vi "Duplicate.vi"(8 "error in":errorcluster, 10 "parameters":variant, 11 "DMM Instrument in":refnum<class "DMM Instrument.lvclass">) -> (0 "error out":errorcluster, 3 "DMM Instrument out":refnum<class "DMM Instrument.lvclass">)   [LabVIEW 2025, in "DMM.lvlib" / "DMM Instrument.lvclass"]
doc: "Implements the specific behavior of a node when it is being duplicated\nCan be used to change the name of the new node for example adding Copy to it. \nCopyright 2017 National Instruments Corporation\n\nLicensed under the Apache License, Version 2.0 (the \"License\"); you may not use this file except in compliance with the License. You may obtain a copy of the License at http://www.apache.org/licenses/LICENSE-2.0\nUnless required by applicable law or agreed to in writing, software distributed under the License is distributed on an \"AS IS\" BASIS, WITHOUT WARRANTIES OR CONDITIONS OF ANY KIND, either express or implied. See the License for the specific language governing permissions and limitations under the License."
uses:
  DMM Instrument.lvclass
  DMM Instrument.lvclass/DMM Instrument.ctl
  DMM configuration/DMM configuration.lvclass
  C:/Users/Public/Documents/Sandia National Labs/TSS Plugin/Abstract Engine.lvlibp/Plugin/Abstract/Instrument configuration/Instrument configuration.lvclass
  Users/Public/Documents/Sandia National Labs/TSS Plugin/Abstract Engine.lvlibp/Plugin/Abstract/Instrument configuration/Read Instrument Setting.vi
  Users/Public/Documents/Sandia National Labs/TSS Plugin/Abstract Engine.lvlibp/Plugin/Abstract/Instrument configuration/Write Instrument Setting.vi
  Users/Public/Documents/Sandia National Labs/TSS Plugin/Abstract Engine.lvlibp/Plugin/Abstract/Abstract Instrument/Abstract Instrument.lvclass
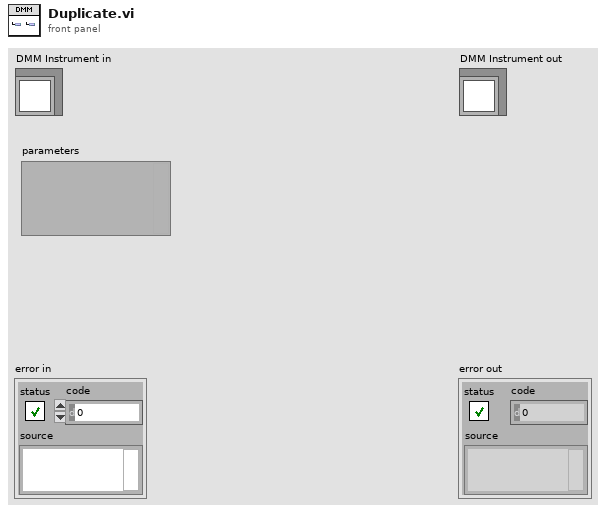
[diagram p1: front panel]
types:
  T1 = typedef "Abstract Engine.lvlibp/Instrument configuration.lvclass/Default Instrument.ctl" = cluster{"Type":string, "Address":string, "SW Alias":string, "Description":string, "Enabled":bool}
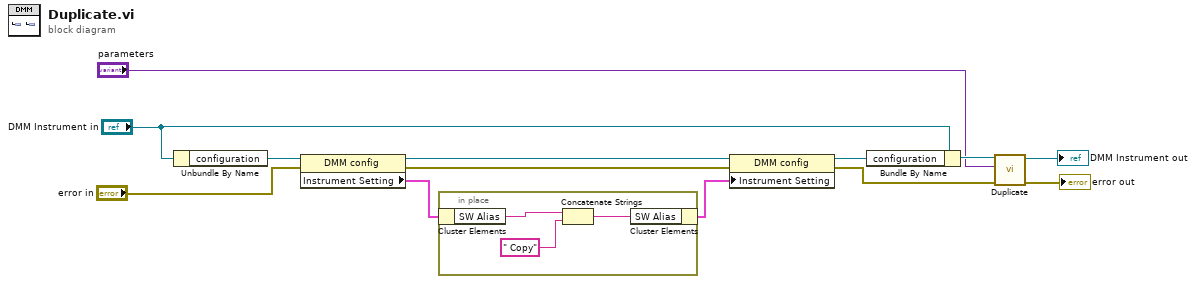
[diagram p0: block diagram]
diagram:
  n1 = Unbundle By Name("DMM Instrument in") -> ("configuration"=w7:refnum<class "DMM configuration.lvclass">)
  n2 = property class="DMM config"(reference=w7, error in="error in") -> (reference out=w6:refnum<class "DMM configuration.lvclass">, error out=w3:errorcluster, "Instrument Setting"=w4:T1)
  n3 = in-place {
    n4 = in-place-cluster #1(w4) -> ("SW Alias"=w16:string)
    n5 = Concatenate Strings(w16, " Copy") -> (w15:string)
    n6 = in-place-cluster #1("SW Alias"=w15) -> (w1:T1)
  }
  n7 = property class="DMM config"(reference=w6, error in=w3, "Instrument Setting"=w1) -> (reference out=w5:refnum<class "DMM configuration.lvclass">, error out=w11:errorcluster)
  n8 = Bundle By Name(cluster="DMM Instrument in", "configuration"=w5) -> (w9:refnum<class "DMM Instrument.lvclass">)
  n9 = call-parent "Duplicate.vi"("error in"=w11, "parameters"="parameters", "CEF_Serialize node in"=w9) -> ("error out"=→"error out":errorcluster, "CEF_Serialize node out"=→"DMM Instrument out":refnum<class "DMM Instrument.lvclass">)  [unwired: 7 in]
